vi "Append Pass-Through Waypoint.vi"(0 "Waypoint Array In":T1[](array[typedef]), 1 "Speed (m/s)":sgl=1.0, 5 "Lat":sgl, 7 "Lon":sgl, 9 "Altitude (m)":sgl, 11 "Error In":errorcluster, 12 "Capture Photo":bool, 13 "Grid Waypoint?":bool, 14 "Capture Time (s)":sgl) -> (4 "appended array":T1[](array[typedef]), 15 "Error Out":errorcluster)   [LabVIEW 2014]
uses:
  Controls/Mission Planning Controls/MAVLINK Mission Item.ctl
  Controls/MAVLINK Mav Frame.ctl
  Commands/Mission Planning/MISSION_ITEM SubVI/MISSION_ITEM Waypoint.vi
  Commands/Mission Planning/MISSION_ITEM SubVI/MISSION_ITEM Set ROI.vi
  Commands/Mission Planning/MISSION_ITEM SubVI/MISSION_ITEM Condition YAW.vi
  Commands/Mission Planning/MISSION_ITEM SubVI/MISSION_ITEM Change Speed.vi
  Commands/Mission Planning/MISSION_ITEM SubVI/MISSION_ITEM Take Photo.vi
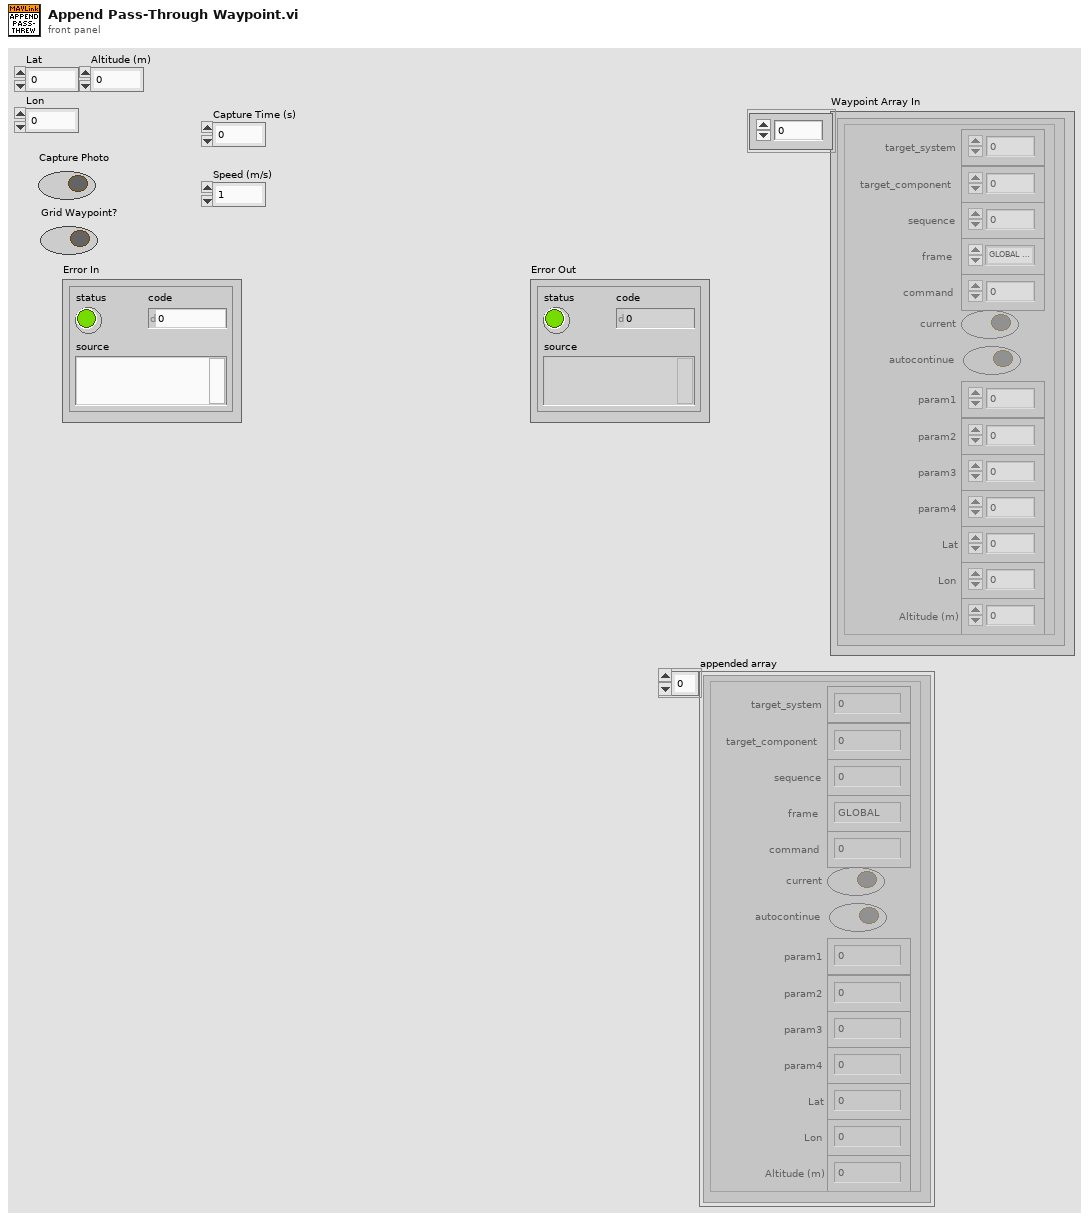
[diagram p1: front panel]
types:
  T1 = typedef "MAVLINK Mission Item.ctl" = cluster{"target_system":u8, "target_component":u8, "sequence":u16, "frame":T2, "command":u16, "current":bool, "autocontinue":bool, "param1":sgl, "param2":sgl, "param3":sgl, "param4":sgl, "Lat":sgl, "Lon":sgl, "Altitude (m)":sgl}
  T2 = typedef "MAVLINK Mav Frame.ctl" = enum8{"GLOBAL", "LOCAL NED", "MISSION", "GLOBAL RELATIVE ALT", "LOCAL ENU", "GLOBAL INT", "GLOBAL RELATIVE ALT INT", "LOCAL OFFSET NED", "BODY NED", "BODY OFFSET NED", "GLOBAL TERRAIN ALT", "GLOBAL TERRAIN ALT INT"}
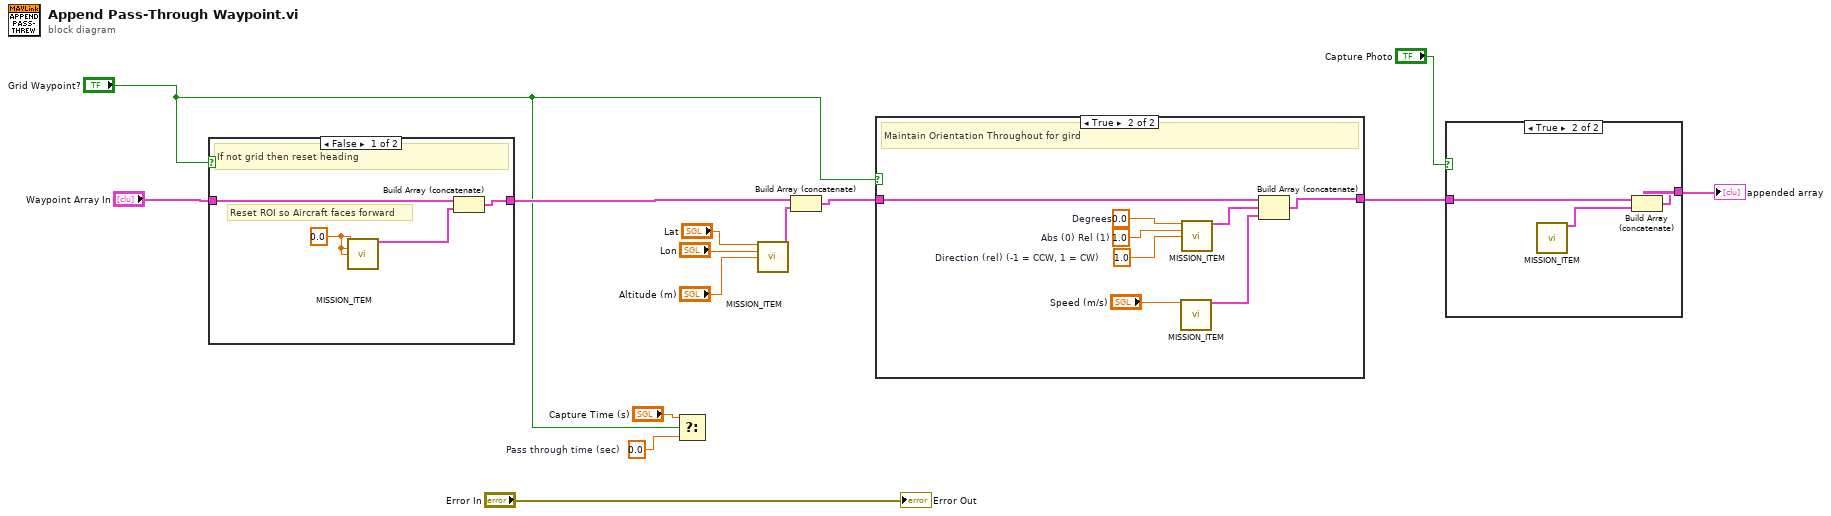
[diagram p0: block diagram]
diagram:
  w4 = sgl 0.0  # Pass through time (sec)
  n1 = case shown="False" "Grid Waypoint?" {
    tunnel: "Waypoint Array In" -> [w17 w19]
    tunnel: [w15 w19] -> w6
    frame False {
      w18 = sgl 0.0 ("Lat")
      # "Reset ROI so Aircraft faces forward"
      # "If not grid then reset heading"
      n2 = call-poly "MISSION_ITEM.vi"("Lat"=w18, "Lon"=w18, "Altitude (m)"=w18) -> ("Mission Item"=w16:T1)  [unwired: 12 in]
      n3 = Build Array (concatenate)(w17, w16) -> (w15:T1[])
    }
    frame True {
      # "Maintain heading for grid waypoint"
    }
  }
  n4 = Select(t="Capture Time (s)", s="Grid Waypoint?", f=w4) -> ()  [unwired: 1 out]
  n5 = call-poly "MISSION_ITEM.vi"("Lat"="Lat", "Lon"="Lon", "Altitude (m)"="Altitude (m)") -> ("Mission Item"=w13:T1)  [unwired: 12 in]
  n6 = Build Array (concatenate)(w6, w13) -> (w8:T1[])
  n7 = case shown="True" "Grid Waypoint?" {
    tunnel: w8 -> [w20 w28]
    tunnel: [w20 w27] -> w3
    frame False {
      # "Not a Grid Waypoint"
    }
    frame True {
      w24 = sgl 1.0  # Direction (rel) (-1 = CCW, 1 = CW)
      w25 = sgl 1.0  # Abs (0) Rel (1)
      w26 = sgl 0.0  # Degrees
      # "Maintain Orientation Throughout for gird"
      n8 = call-poly "MISSION_ITEM.vi"("Speed (m/s)"="Speed (m/s)") -> ("Mission Item"=w22:T1)  [unwired: 14 in]
      n9 = call-poly "MISSION_ITEM.vi"("Degrees"=w26, "Abs (0) Rel (1)"=w25, "Direction (rel) (-1 = CCW, 1 = CW)"=w24) -> ("Mission Item"=w23:T1)  [unwired: 12 in]
      n10 = Build Array (concatenate)(w28, w23, w22) -> (w27:T1[])
    }
  }
  n11 = case shown="True" "Capture Photo" {
    tunnel: w3 -> [w29 w32]
    tunnel: [w29 w31] -> w9
    frame False {
    }
    frame True {
      n12 = call-poly "MISSION_ITEM.vi"() -> ("Mission Item"=w30:T1)  [unwired: 15 in]
      n13 = Build Array (concatenate)(w32, w30) -> (w31:T1[])
    }
  }
  "appended array" <- w9
  "Error Out" <- "Error In"
